vi "Weather Parse Test.vi"() -> ()   [LabVIEW 2020, in "CDM-Config.lvlib"] (continued)
\"2025-12-02T17:12:00-07:00\"\n                    }\n                ],\n                \"sent\": \"2025-12-03T02:08:00-07:00\",\n                \"effective\": \"2025-12-03T02:08:00-07:00\",\n                \"onset\": \"2025-12-03T02:08:00-07:00\",\n                \"expires\": \"2025-12-03T17:00:00-07:00\",\n                \"ends\": \"2025-12-04T02:00:00-07:00\",\n                \"status\": \"Actual\",\n                \"messageType\": \"Update\",\n                \"category\": \"Met\",\n                \"severity\": \"Moderate\",\n                \"certainty\": \"Likely\",\n                \"urgency\": \"Expected\",\n                \"event\": \"Winter Weather Advisory\",\n                \"sender\": \"w-nws.webmaster@noaa.gov\",\n                \"senderName\": \"NWS Grand Junction CO\",\n                \"headline\": \"Winter Weather Advisory issued December 3 at 2:08AM MST until December 4 at 2:00AM MST by NWS Grand Junction CO\",\n                \"description\": \"* WHAT...Snow. Total snow accumulations between 6 and 10 inches with\\nlocally higher amounts.\\n\\n* WHERE...Southwest San Juan Mountains.\\n\\n* WHEN...Until 2 AM MST Thursday.\\n\\n* IMPACTS...Travel could be very difficult. The hazardous conditions\\ncould impact the Wednesday morning and evening commutes.\",\n                \"instruction\": \"Slow down and use caution while traveling. The latest road\\nconditions for the state you are calling from can be obtained by\\ncalling 5 1 1.\",\n                \"response\": \"Execute\",\n                \"parameters\": {\n                    \"AWIPSidentifier\": [\n                        \"WSWGJT\"\n                    ],\n                    \"WMOidentifier\": [\n                        \"WWUS45 KGJT 030908\"\n                    ],\n                    \"NWSheadline\": [\n                        \"WINTER WEATHER ADVISORY REMAINS IN EFFECT UNTIL 2 AM MST THURSDAY\"\n                    ],\n                    \"BLOCKCHANNEL\": [\n                        \"EAS\",\n                        \"NWEM\",\n                        \"CMAS\"\n                    ],\n                    \"VTEC\": [\n                        \"/O.CON.KGJT.WW.Y.0026.000000T0000Z-251204T0900Z/\"\n                    ],\n                    \"eventEndingTime\": [\n                        \"2025-12-04T02:00:00-07:00\"\n                    ]\n                },\n                \"scope\": \"Public\",\n                \"code\": \"IPAWSv1.0\",\n                \"language\": \"en-US\",\n                \"web\": \"http://www.weather.gov\",\n                \"eventCode\": {\n                    \"SAME\": [\n                        \"NWS\"\n                    ],\n                    \"NationalWeatherService\": [\n                        \"WWY\"\n                    ]\n                }\n            }\n        },\n        {\n            \"id\": \"https://api.weather.gov/alerts/urn:oid:2.49.0.1.840.0.ecc18ad1715ddd59d073d3396e68cd94d8156f26.002.1\",\n            \"type\": \"Feature\",\n            \"geometry\": null,\n            \"properties\": {\n                \"@id\": \"https://api.weather.gov/alerts/urn:oid:2.49.0.1.840.0.ecc18ad1715ddd59d073d3396e68cd94d8156f26.002.1\",\n                \"@type\": \"wx:Alert\",\n                \"id\": \"urn:oid:2.49.0.1.840.0.ecc18ad1715ddd59d073d3396e68cd94d8156f26.002.1\",\n                \"areaDesc\": \"Elkhead and Park Mountains; Gore and Elk Mountains/Central Mountain Valleys\",\n                \"geocode\": {\n                    \"SAME\": [\n                        \"008081\",\n                        \"008107\",\n                        \"008037\",\n                        \"008045\",\n                        \"008097\"\n                    ],\n                    \"UGC\": [\n                        \"COZ004\",\n                        \"COZ010\"\n                    ]\n                },\n                \"affectedZones\": [\n                    \"https://api.weather.gov/zones/forecast/COZ004\",\n                    \"https://api.weather.gov/zones/forecast/COZ010\"\n                ],\n                \"references\": [\n                    {\n                        \"@id\": \"https://api.weather.gov/alerts/urn:oid:2.49.0.1.840.0.59f7bbb1b05f341c96e55d508e395b781ba80eb6.003.1\",\n                        \"identifier\": \"urn:oid:2.49.0.1.840.0.59f7bbb1b05f341c96e55d508e395b781ba80eb6.003.1\",\n                        \"sender\": \"w-nws.webmaster@noaa.gov\",\n                        \"sent\": \"2025-12-02T12:59:00-07:00\"\n                    },\n                    {\n                        \"@id\": \"https://api.weather.gov/alerts/urn:oid:2.49.0.1.840.0.1e2e3f318117076bbf552163bdfe24a72a2e2d99.002.1\",\n                        \"identifier\": \"urn:oid:2.49.0.1.840.0.1e2e3f318117076bbf552163bdfe24a72a2e2d99.002.1\",\n                        \"sender\": \"w-nws.webmaster@noaa.gov\",\n                        \"sent\": \"2025-12-02T17:12:00-07:00\"\n                    }\n                ],\n                \"sent\": \"2025-12-03T02:08:00-07:00\",\n                \"effective\": \"2025-12-03T02:08:00-07:00\",\n                \"onset\": \"2025-12-03T02:08:00-07:00\",\n                \"expires\": \"2025-12-03T17:00:00-07:00\",\n                \"ends\": \"2025-12-03T17:00:00-07:00\",\n                \"status\": \"Actual\",\n                \"messageType\": \"Update\",\n                \"category\": \"Met\",\n                \"severity\": \"Moderate\",\n                \"certainty\": \"Likely\",\n                \"urgency\": \"Expected\",\n                \"event\": \"Winter Weather Advisory\",\n                \"sender\": \"w-nws.webmaster@noaa.gov\",\n                \"senderName\": \"NWS Grand Junction CO\",\n                \"headline\": \"Winter Weather Advisory issued December 3 at 2:08AM MST until December 3 at 5:00PM MST by NWS Grand Junction CO\",\n                \"description\": \"* WHAT...Snow. Additional snow accumulations between 2 and 4 inches.\\n\\n* WHERE...Elkhead and Park Mountains, Northwest San Juan Mountains,\\nand Gore and Elk Mountains/Central Mountain Valleys.\\n\\n* WHEN...Until 5 PM MST this afternoon.\\n\\n* IMPACTS...Roads, and especially bridges and overpasses, will\\nlikely become slick and hazardous. Plan on slippery road\\nconditions. The hazardous conditions could impact the Wednesday\\nmorning and evening commutes.\",\n                \"instruction\": \"Slow down and use caution while traveling. The latest road\\nconditions for the state you are calling from can be obtained by\\ncalling 5 1 1.\",\n                \"response\": \"Execute\",\n                \"parameters\": {\n                    \"AWIPSidentifier\": [\n                        \"WSWGJT\"\n                    ],\n                    \"WMOidentifier\": [\n                        \"WWUS45 KGJT 030908\"\n                    ],\n                    \"NWSheadline\": [\n                        \"WINTER WEATHER ADVISORY REMAINS IN EFFECT UNTIL 5 PM MST THIS AFTERNOON\"\n                    ],\n                    \"BLOCKCHANNEL\": [\n                        \"EAS\",\n                        \"NWEM\",\n                        \"CMAS\"\n                    ],\n                    \"VTEC\": [\n                        \"/O.CON.KGJT.WW.Y.0026.000000T0000Z-251204T0000Z/\"\n                    ],\n                    \"eventEndingTime\": [\n                        \"2025-12-03T17:00:00-07:00\"\n                    ],\n                    \"expiredReferences\": [\n                        \"w-nws.webmaster@noaa.gov,urn:oid:2.49.0.1.840.0.679f6cdd98833ec879584b0a7abc7307ca2a58e6.001.1,2025-12-02T02:26:00-07:00\"\n                    ]\n                },\n                \"scope\": \"Public\",\n                \"code\": \"IPAWSv1.0\",\n                \"language\": \"en-US\",\n                \"web\": \"http://www.weather.gov\",\n                \"eventCode\": {\n                    \"SAME\": [\n                        \"NWS\"\n                    ],\n                    \"NationalWeatherService\": [\n                        \"WWY\"\n                    ]\n                }\n            }\n        },\n        {\n            \"id\": \"https://api.weather.gov/alerts/urn:oid:2.49.0.1.840.0.ecc18ad1715ddd59d073d3396e68cd94d8156f26.004.1\",\n            \"type\": \"Feature\",\n            \"geometry\": null,\n            \"properties\": {\n                \"@id\": \"https://api.weather.gov/alerts/urn:oid:2.49.0.1.840.0.ecc18ad1715ddd59d073d3396e68cd94d8156f26.004.1\",\n                \"@type\": \"wx:Alert\",\n                \"id\": \"urn:oid:2.49.0.1.840.0.ecc18ad1715ddd59d073d3396e68cd94d8156f26.004.1\",\n                \"areaDesc\": \"Northwestern San Juan Mountains\",\n                \"geocode\": {\n                    \"SAME\": [\n                        \"008051\",\n                        \"008053\",\n                        \"008085\",\n                        \"008091\",\n                        \"008113\"\n                    ],\n                    \"UGC\": [\n                        \"COZ018\"\n                    ]\n                },\n                \"affectedZones\": [\n                    \"https://api.weather.gov/zones/forecast/COZ018\"\n                ],\n                \"references\": [\n                    {\n                        \"@id\": \"https://api.weather.gov/alerts/urn:oid:2.49.0.1.840.0.59f7bbb1b05f341c96e55d508e395b781ba80eb6.002.1\",\n                        \"identifier\": \"urn:oid:2.49.0.1.840.0.59f7bbb1b05f341c96e55d508e395b781ba80eb6.002.1\",\n                        \"sender\": \"w-nws.webmaster@noaa.gov\",\n                        \"sent\": \"2025-12-02T12:59:00-07:00\"\n                    },\n                    {\n                        \"@id\": \"https://api.weather.gov/alerts/urn:oid:2.49.0.1.840.0.1e2e3f318117076bbf552163bdfe24a72a2e2d99.003.1\",\n                        \"identifier\": \"urn:oid:2.49.0.1.840.0.1e2e3f318117076bbf552163bdfe24a72a2e2d99.003.1\",\n                        \"sender\": \"w-nws.webmaster@noaa.gov\",\n                        \"sent\": \"2025-12-02T17:12:00-07:00\"\n                    }\n                ],\n                \"sent\": \"2025-12-03T02:08:00-07:00\",\n                \"effective\": \"2025-12-03T02:08:00-07:00\",\n                \"onset\": \"2025-12-03T02:08:00-07:00\",\n                \"expires\": \"2025-12-03T17:00:00-07:00\",\n                \"ends\": \"2025-12-04T02:00:00-07:00\",\n                \"status\": \"Actual\",\n                \"messageType\": \"Update\",\n                \"category\": \"Met\",\n                \"severity\": \"Moderate\",\n                \"certainty\": \"Likely\",\n                \"urgency\": \"Expected\",\n                \"event\": \"Winter Weather Advisory\",\n                \"sender\": \"w-nws.webmaster@noaa.gov\",\n                \"senderName\": \"NWS Grand Junction CO\",\n                \"headline\": \"Winter Weather Advisory issued December 3 at 2:08AM MST until December 4 at 2:00AM MST by NWS Grand Junction CO\",\n                \"description\": \"* WHAT...Snow. Total snow accumulations between 6 and 10 inches with\\nlocally higher amounts.\\n\\n* WHERE...Northwest San Juan Mountains.\\n\\n* WHEN...Until 2 AM MST Thursday.\\n\\n* IMPACTS...Travel could be very difficult. The hazardous conditions\\ncould impact the Wednesday morning and evening commutes.\",\n                \"instruction\": \"Slow down and use caution while traveling. The latest road\\nconditions for the state you are calling from can be obtained by\\ncalling 5 1 1.\",\n                \"response\": \"Execute\",\n                \"parameters\": {\n                    \"AWIPSidentifier\": [\n                        \"WSWGJT\"\n                    ],\n                    \"WMOidentifier\": [\n                        \"WWUS45 KGJT 030908\"\n                    ],\n                    \"NWSheadline\": [\n                        \"WINTER WEATHER ADVISORY REMAINS IN EFFECT UNTIL 2 AM MST THURSDAY\"\n                    ],\n                    \"BLOCKCHANNEL\": [\n                        \"EAS\",\n                        \"NWEM\",\n                        \"CMAS\"\n                    ],\n                    \"VTEC\": [\n                        \"/O.CON.KGJT.WW.Y.0026.000000T0000Z-251204T0900Z/\"\n                    ],\n                    \"eventEndingTime\": [\n                        \"2025-12-04T02:00:00-07:00\"\n                    ],\n                    \"expiredReferences\": [\n                        \"w-nws.webmaster@noaa.gov,urn:oid:2.49.0.1.840.0.679f6cdd98833ec879584b0a7abc7307ca2a58e6.001.1,2025-12-02T02:26:00-07:00\"\n                    ]\n                },\n                \"scope\": \"Public\",\n                \"code\": \"IPAWSv1.0\",\n                \"language\": \"en-US\",\n                \"web\": \"http://www.weather.gov\",\n                \"eventCode\": {\n                    \"SAME\": [\n                        \"NWS\"\n                    ],\n                    \"NationalWeatherService\": [\n                        \"WWY\"\n                    ]\n                }\n            }\n        },\n        {\n            \"id\": \"https://api.weather.gov/alerts/urn:oid:2.49.0.1.840.0.e71cf2b83fde77384319b715682951004f37611d.001.2\",\n            \"type\": \"Feature\",\n            \"geometry\": null,\n            \"properties\": {\n                \"@id\": \"https://api.weather.gov/alerts/urn:oid:2.49.0.1.840.0.e71cf2b83fde77384319b715682951004f37611d.001.2\",\n                \"@type\": \"wx:Alert\",\n                \"id\": \"urn:oid:2.49.0.1.840.0.e71cf2b83fde77384319b715682951004f37611d.001.2\",\n                \"areaDesc\": \"Rock Island Passage to Sturgeon Bay WI\",\n                \"geocode\": {\n                    \"SAME\": [\n                        \"092541\"\n                    ],\n                    \"UGC\": [\n                        \"LMZ541\"\n                    ]\n                },\n                \"affectedZones\": [\n                    \"https://api.weather.gov/zones/forecast/LMZ541\"\n                ],\n                \"references\": [],\n                \"sent\": \"2025-12-03T03:06:00-06:00\",\n                \"effective\": \"2025-12-03T03:06:00-06:00\",\n                \"onset\": \"2025-12-04T21:00:00-06:00\",\n                \"expires\": \"2025-12-03T11:15:00-06:00\",\n                \"ends\": \"2025-12-05T06:00:00-06:00\",\n                \"status\": \"Actual\",\n                \"messageType\": \"Alert\",\n                \"category\": \"Met\",\n                \"severity\": \"Moderate\",\n                \"certainty\": \"Possible\",\n                \"urgency\": \"Future\",\n                \"event\": \"Gale Watch\",\n                \"sender\": \"w-nws.webmaster@noaa.gov\",\n                \"senderName\": \"NWS Green Bay WI\",\n                \"headline\": \"Gale Watch issued December 3 at 3:06AM CST until December 5 at 6:00AM CST by NWS Green Bay WI\",\n                \"description\": \"* WHAT...For the Small Craft Advisory, northwest winds 15 to 20\\nkt with gusts up to 25 kt and waves 2 to 5 ft. For the Gale\\nWatch, southwest winds 20 to 25 kt with gusts up to 35 kt and\\nwaves 4 to 7 ft possible.\\n\\n* WHERE...Lake Michigan nearshore waters from Washington Island\\nto Sturgeon Bay.\\n\\n* WHEN...For the Small Craft Advisory, until 3 AM CST Thursday.\\nFor the Gale Watch, from Thursday evening through late\\nThursday night.\\n\\n* IMPACTS...Strong winds can cause hazardous waves which could\\ncapsize or damage vessels and reduce visibility.\",\n                \"instruction\": \"Mariners should consider altering plans to avoid possible\\nhazardous conditions.  Remain in port, seek safe harbor, alter\\ncourse, and/or secure the vessel for severe wind and waves.\",\n                \"response\": \"Prepare\",\n                \"parameters\": {\n                    \"AWIPSidentifier\": [\n                        \"MWWGRB\"\n                    ],\n                    \"WMOidentifier\": [\n                        \"WHUS73 KGRB 030906\"\n                    ],\n                    \"NWSheadline\": [\n                        \"SMALL CRAFT ADVISORY REMAINS IN EFFECT UNTIL 3 AM CST THURSDAY... ...GALE WATCH IN EFFECT FROM THURSDAY EVENING THROUGH LATE THURSDAY NIGHT\"\n                    ],\n                    \"BLOCKCHANNEL\": [\n                        \"EAS\",\n                        \"NWEM\",\n                        \"CMAS\"\n                    ],\n                    \"VTEC\": [\n                        \"/O.NEW.KGRB.GL.A.0006.251205T0300Z-251205T1200Z/\"\n                    ],\n                    \"eventEndingTime\": [\n                        \"2025-12-05T06:00:00-06:00\"\n                    ]\n                },\n                \"scope\": \"Public\",\n                \"code\": \"IPAWSv1.0\",\n                \"language\": \"en-US\",\n                \"web\": \"http://www.weather.gov\",\n                \"eventCode\": {\n                    \"SAME\": [\n                        \"NWS\"\n                    ],\n                    \"NationalWeatherService\": [\n                        \"GLA\"\n                    ]\n                }\n            }\n        },\n        {\n            \"id\": \"https://api.weather.gov/alerts/urn:oid:2.49.0.1.840.0.e71cf2b83fde77384319b715682951004f37611d.002.2\",\n            \"type\": \"Feature\",\n            \"geometry\": null,\n            \"properties\": {\n                \"@id\": \"https://api.weather.gov/alerts/urn:oid:2.49.0.1.840.0.e71cf2b83fde77384319b715682951004f37611d.002.2\",\n                \"@type\": \"wx:Alert\",\n                \"id\": \"urn:oid:2.49.0.1.840.0.e71cf2b83fde77384319b715682951004f37611d.002.2\",\n                \"areaDesc\": \"Green Bay south of line from  Cedar River to Rock Island Passage and north of a line from Oconto WI to Little Sturgeon Bay WI\",\n                \"geocode\": {\n                    \"SAME\": [\n                        \"092521\"\n                    ],\n                    \"UGC\": [\n                        \"LMZ521\"\n                    ]\n                },\n                \"affectedZones\": [\n                    \"https://api.weather.gov/zones/forecast/LMZ521\"\n                ],\n                \"references\": [],\n                \"sent\": \"2025-12-03T03:06:00-06:00\",\n                \"effective\": \"2025-12-03T03:06:00-06:00\",\n                \"onset\": \"2025-12-04T21:00:00-06:00\",\n                \"expires\": \"2025-12-03T11:15:00-06:00\",\n                \"ends\": \"2025-12-05T06:00:00-06:00\",\n                \"status\": \"Actual\",\n                \"messageType\": \"Alert\",\n                \"category\": \"Met\",\n                \"severity\": \"Moderate\",\n                \"certainty\": \"Possible\",\n                \"urgency\": \"Future\",\n                \"event\": \"Gale Watch\",\n                \"sender\": \"w-nws.webmaster@noaa.gov\",\n                \"senderName\": \"NWS Green Bay WI\",\n                \"headline\": \"Gale Watch issued December 3 at 3:06AM CST until December 5 at 6:00AM CST by NWS Green Bay WI\",\n                \"description\": \"* WHAT...For the Small Craft Advisory, northwest winds 15 to 25\\nkt and waves 1 to 4 ft. For the Gale Watch, southwest winds 20\\nto 25 kt with gusts up to 35 kt and waves 5 to 8 ft possible.\\n\\n* WHERE...Central Bay of Green Bay.\\n\\n* WHEN...For the Small Craft Advisory, until 3 AM CST Thursday.\\nFor the Gale Watch, from Thursday evening through late\\nThursday night.\\n\\n* IMPACTS...Strong winds can cause hazardous waves which could\\ncapsize or damage vessels and reduce visibility.\",\n                \"instruction\": \"Mariners should consider altering plans to avoid possible\\nhazardous conditions.  Remain in port, seek safe harbor, alter\\ncourse, and/or secure the vessel for severe wind and waves.\",\n                \"response\": \"Prepare\",\n                \"parameters\": {\n                    \"AWIPSidentifier\": [\n                        \"MWWGRB\"\n                    ],\n                    \"WMOidentifier\": [\n                        \"WHUS73 KGRB 030906\"\n                    ],\n                    \"NWSheadline\": [\n                        \"SMALL CRAFT ADVISORY REMAINS IN EFFECT UNTIL 3 AM CST THURSDAY... ...GALE WATCH IN EFFECT FROM THURSDAY EVENING THROUGH LATE THURSDAY NIGHT\"\n                    ],\n                    \"BLOCKCHANNEL\": [\n                        \"EAS\",\n                        \"NWEM\",\n                        \"CMAS\"\n                    ],\n                    \"VTEC\": [\n                        \"/O.NEW.KGRB.GL.A.0006.251205T0300Z-251205T1200Z/\"\n                    ],\n                    \"eventEndingTime\": [\n                        \"2025-12-05T06:00:00-06:00\"\n                    ]\n                },\n                \"scope\": \"Public\",\n                \"code\": \"IPAWSv1.0\",\n                \"language\": \"en-US\",\n                \"web\": \"http://www.weather.gov\",\n                \"eventCode\": {\n                    \"SAME\": [\n                        \"NWS\"\n                    ],\n                    \"NationalWeatherService\": [\n                        \"GLA\"\n                    ]\n                }\n            }\n        },\n        {\n            \"id\": \"https://api.weather.gov/alerts/urn:oid:2.49.0.1.840.0.e71cf2b83fde77384319b715682951004f37611d.002.1\",\n            \"type\": \"Feature\",\n            \"geometry\": null,\n            \"properties\": {\n                \"@id\": \"https://api.weather.gov/alerts/urn:oid:2.49.0.1.840.0.e71cf2b83fde77384319b715682951004f37611d.002.1\",\n                \"@type\": \"wx:Alert\",\n                \"id\": \"urn:oid:2.49.0.1.840.0.e71cf2b83fde77384319b715682951004f37611d.002.1\",\n                \"areaDesc\": \"Green Bay south of line from  Cedar River to Rock Island Passage and north of a line from Oconto WI to Little Sturgeon Bay WI\",\n                \"geocode\": {\n                    \"SAME\": [\n                        \"092521\"\n                    ],\n                    \"UGC\": [\n                        \"LMZ521\"\n                    ]\n                },\n                \"affectedZones\": [\n                    \"https://api.weather.gov/zones/forecast/LMZ521\"\n                ],\n                \"references\": [\n                    {\n                        \"@id\": \"https://api.weather.gov/alerts/urn:oid:2.49.0.1.840.0.769b5a057bb88d56f701a5e0b04efae8c3b52336.002.1\",\n                        \"identifier\": \"urn:oid:2.49.0.1.840.0.769b5a057bb88d56f701a5e0b04efae8c3b52336.002.1\",\n                        \"sender\": \"w-nws.webmaster@noaa.gov\",\n                        \"sent\": \"2025-12-02T21:04:00-06:00\"\n                    }\n                ],\n                \"sent\": \"2025-12-03T03:06:00-06:00\",\n                \"effective\": \"2025-12-03T03:06:00-06:00\",\n                \"onset\": \"2025-12-03T03:06:00-06:00\",\n                \"expires\": \"2025-12-03T11:15:00-06:00\",\n                \"ends\": \"2025-12-04T03:00:00-06:00\",\n                \"status\": \"Actual\",\n                \"messageType\": \"Update\",\n                \"category\": \"Met\",\n                \"severity\": \"Minor\",\n                \"certainty\": \"Likely\",\n                \"urgency\": \"Expected\",\n                \"event\": \"Small Craft Advisory\",\n                \"sender\": \"w-nws.webmaster@noaa.gov\",\n                \"senderName\": \"NWS Green Bay WI\",\n                \"headline\": \"Small Craft Advisory issued December 3 at 3:06AM CST until December 4 at 3:00AM CST by NWS Green Bay WI\",\n                \"description\": \"* WHAT...For the Small Craft Advisory, northwest winds 15 to 25\\nkt and waves 1 to 4 ft. For the Gale Watch, southwest winds 20\\nto 25 kt with gusts up to 35 kt and waves 5 to 8 ft possible.\\n\\n* WHERE...Central Bay of Green Bay.\\n\\n* WHEN...For the Small Craft Advisory, until 3 AM CST Thursday.\\nFor the Gale Watch, from Thursday evening through late\\nThursday night.\\n\\n* IMPACTS...Strong winds can cause hazardous waves which could\\ncapsize or damage vessels and reduce visibility.\",\n                \"instruction\": \"Mariners should consider altering plans to avoid possible\\nhazardous conditions.  Remain in port, seek safe harbor, alter\\ncourse, and/or secure the vessel for severe wind and waves.\",\n                \"response\": \"Avoid\",\n                \"parameters\": {\n                    \"AWIPSidentifier\": [\n                        \"MWWGRB\"\n                    ],\n                    \"WMOidentifier\": [\n                        \"WHUS73 KGRB 030906\"\n                    ],\n                    \"NWSheadline\": [\n                        \"SMALL CRAFT ADVISORY REMAINS IN EFFECT UNTIL 3 AM CST THURSDAY... ...GALE WATCH IN EFFECT FROM THURSDAY EVENING THROUGH LATE THURSDAY NIGHT\"\n                    ],\n                    \"BLOCKCHANNEL\": [\n                        \"EAS\",\n                        \"NWEM\",\n                        \"CMAS\"\n                    ],\n                    \"VTEC\": [\n                        \"/O.CON.KGRB.SC.Y.0092.000000T0000Z-251204T0900Z/\"\n                    ],\n                    \"eventEndingTime\": [\n                        \"2025-12-04T03:00:00-06:00\"\n                    ],\n                    \"expiredReferences\": [\n                        \"w-nws.webmaster@noaa.gov,urn:oid:2.49.0.1.840.0.4daec37cfaba31be0f4161c4db8c289fd8fca270.002.1,2025-12-02T16:20:00-06:00 w-nws.webmaster@noaa.gov,urn:oid:2.49.0.1.840.0.22088d8fd19601efe26ef283f0aea20a6c82bd22.002.1,2025-12-02T10:40:00-06:00 w-nws.webmaster@noaa.gov,urn:oid:2.49.0.1.840.0.4d26ff1add25a90f0bbaf88a1a22cd2917cf1fd9.002.1,2025-12-02T03:00:00-06:00\"\n                    ]\n                },\n                \"scope\": \"Public\",\n                \"code\": \"IPAWSv1.0\",\n                \"language\": \"en-US\",\n                \"web\": \"http://www.weather.gov\",\n                \"eventCode\": {\n                    \"SAME\": [\n                        \"NWS\"\n                    ],\n                    \"NationalWeatherService\": [\n                        \"SCY\"\n                    ]\n                }\n            }\n        },\n        {\n            \"id\": \"https://api.weather.gov/alerts/urn:oid:2.49.0.1.840.0.e71cf2b83fde77384319b715682951004f37611d.004.1\",\n            \"type\": \"Feature\",\n            \"geometry\": null,\n            \"properties\": {\n                \"@id\": \"https://api.weather.gov/alerts/urn:oid:2.49.0.1.840.0.e71cf2b83fde77384319b715682951004f37611d.004.1\",\n                \"@type\": \"wx:Alert\",\n                \"id\": \"urn:oid:2.49.0.1.840.0.e71cf2b83fde77384319b715682951004f37611d.004.1\",\n                \"areaDesc\": \"Green Bay south of line from  Oconto WI to Little Sturgeon Bay WI\",\n                \"geocode\": {\n                    \"SAME\": [\n                        \"092522\"\n                    ],\n                    \"UGC\": [\n                        \"LMZ522\"\n                    ]\n                },\n                \"affectedZones\": [\n                    \"https://api.weather.gov/zones/forecast/LMZ522\"\n                ],\n                \"references\": [\n                    {\n                        \"@id\": \"https://api.weather.gov/alerts/urn:oid:2.49.0.1.840.0.769b5a057bb88d56f701a5e0b04efae8c3b52336.002.1\",\n                        \"identifier\": \"urn:oid:2.49.0.1.840.0.769b5a057bb88d56f701a5e0b04efae8c3b52336.002.1\",\n                        \"sender\": \"w-nws.webmaster@noaa.gov\",\n                        \"sent\": \"2025-12-02T21:04:00-06:00\"\n                    }\n                ],\n                \"sent\": \"2025-12-03T03:06:00-06:00\",\n                \"effective\": \"2025-12-03T03:06:00-06:00\",\n                \"onset\": \"2025-12-03T03:06:00-06:00\",\n                \"expires\": \"2025-12-03T11:15:00-06:00\",\n                \"ends\": \"2025-12-04T03:00:00-06:00\",\n                \"status\": \"Actual\",\n                \"messageType\": \"Update\",\n                \"category\": \"Met\",\n                \"severity\": \"Minor\",\n                \"certainty\": \"Likely\",\n                \"urgency\": \"Expected\",\n                \"event\": \"Small Craft Advisory\",\n                \"sender\": \"w-nws.webmaster@noaa.gov\",\n                \"senderName\": \"NWS Green Bay WI\",\n                \"headline\": \"Small Craft Advisory issued December 3 at 3:06AM CST until December 4 at 3:00AM CST by NWS Green Bay WI\",\n                \"description\": \"* WHAT...Northwest winds 15 to 25 kt and waves 1 to 3 ft.\\n\\n* WHERE...Southern Bay of Green Bay.\\n\\n* WHEN...Until 3 AM CST Thursday.\\n\\n* IMPACTS...Conditions will be hazardous to small craft.\",\n                \"instruction\": \"Inexperienced mariners, especially those operating smaller\\nvessels, should avoid navigating in hazardous conditions.\",\n                \"response\": \"Avoid\",\n                \"parameters\": {\n                    \"AWIPSidentifier\": [\n                        \"MWWGRB\"\n                    ],\n                    \"WMOidentifier\": [\n                        \"WHUS73 KGRB 030906\"\n                    ],\n                    \"NWSheadline\": [\n                        \"SMALL CRAFT ADVISORY REMAINS IN EFFECT UNTIL 3 AM CST THURSDAY\"\n                    ],\n                    \"BLOCKCHANNEL\": [\n                        \"EAS\",\n                        \"NWEM\",\n                        \"CMAS\"\n                    ],\n                    \"VTEC\": [\n                        \"/O.CON.KGRB.SC.Y.0092.000000T0000Z-251204T0900Z/\"\n                    ],\n                    \"eventEndingTime\": [\n                        \"2025-12-04T03:00:00-06:00\"\n                    ],\n                    \"expiredReferences\": [\n                        \"w-nws.webmaster@noaa.gov,urn:oid:2.49.0.1.840.0.4daec37cfaba31be0f4161c4db8c289fd8fca270.002.1,2025-12-02T16:20:00-06:00 w-nws.webmaster@noaa.gov,urn:oid:2.49.0.1.840.0.22088d8fd19601efe26ef283f0aea20a6c82bd22.002.1,2025-12-02T10:40:00-06:00 w-nws.webmaster@noaa.gov,urn:oid:2.49.0.1.840.0.4d26ff1add25a90f0bbaf88a1a22cd2917cf1fd9.002.1,2025-12-02T03:00:00-06:00\"\n                    ]\n                },\n                \"scope\": \"Public\",\n                \"code\": \"IPAWSv1.0\",\n                \"language\": \"en-US\",\n                \"web\": \"http://www.weather.gov\",\n                \"eventCode\": {\n                    \"SAME\": [\n                        \"NWS\"\n                    ],\n                    \"NationalWeatherService\": [\n                        \"SCY\"\n                    ]\n                }\n            }\n        },\n        {\n            \"id\": \"https://api.weather.gov/alerts/urn:oid:2.49.0.1.840.0.e71cf2b83fde77384319b715682951004f37611d.001.1\",\n            \"type\": \"Feature\",\n            \"geometry\": null,\n            \"properties\": {\n                \"@id\": \"https://api.weather.gov/alerts/urn:oid:2.49.0.1.840.0.e71cf2b83fde77384319b715682951004f37611d.001.1\",\n                \"@type\": \"wx:Alert\",\n                \"id\": \"urn:oid:2.49.0.1.840.0.e71cf2b83fde77384319b715682951004f37611d.001.1\",\n                \"areaDesc\": \"Rock Island Passage to Sturgeon Bay WI\",\n                \"geocode\": {\n                    \"SAME\": [\n                        \"092541\"\n                    ],\n                    \"UGC\": [\n                        \"LMZ541\"\n                    ]\n                },\n                \"affectedZones\": [\n                    \"https://api.weather.gov/zones/forecast/LMZ541\"\n                ],\n                \"references\": [\n                    {\n                        \"@id\": \"https://api.weather.gov/alerts/urn:oid:2.49.0.1.840.0.769b5a057bb88d56f701a5e0b04efae8c3b52336.001.1\",\n                        \"identifier\": \"urn:oid:2.49.0.1.840.0.769b5a057bb88d56f701a5e0b04efae8c3b52336.001.1\",\n                        \"sender\": \"w-nws.webmaster@noaa.gov\",\n                        \"sent\": \"2025-12-02T21:04:00-06:00\"\n                    }\n                ],\n                \"sent\": \"2025-12-03T03:06:00-06:00\",\n                \"effective\": \"2025-12-03T03:06:00-06:00\",\n                \"onset\": \"2025-12-03T03:06:00-06:00\",\n                \"expires\": \"2025-12-03T11:15:00-06:00\",\n                \"ends\": \"2025-12-04T03:00:00-06:00\",\n                \"status\": \"Actual\",\n                \"messageType\": \"Update\",\n                \"category\": \"Met\",\n                \"severity\": \"Minor\",\n                \"certainty\": \"Likely\",\n                \"urgency\": \"Expected\",\n                \"event\": \"Small Craft Advisory\",\n                \"sender\": \"w-nws.webmaster@noaa.gov\",\n                \"senderName\": \"NWS Green Bay WI\",\n                \"headline\": \"Small Craft Advisory issued December 3 at 3:06AM CST until December 4 at 3:00AM CST by NWS Green Bay WI\",\n                \"description\": \"* WHAT...For the Small Craft Advisory, northwest winds 15 to 20\\nkt with gusts up to 25 kt and waves 2 to 5 ft. For the Gale\\nWatch, southwest winds 20 to 25 kt with gusts up to 35 kt and\\nwaves 4 to 7 ft possible.\\n\\n* WHERE...Lake Michigan nearshore waters from Washington Island\\nto Sturgeon Bay.\\n\\n* WHEN...For the Small Craft Advisory, until 3 AM CST Thursday.\\nFor the Gale Watch, from Thursday evening through late\\nThursday night.\\n\\n* IMPACTS...Strong winds can cause hazardous waves which could\\ncapsize or damage vessels and reduce visibility.\",\n                \"instruction\": \"Mariners should consider altering plans to avoid possible\\nhazardous conditions.  Remain in port, seek safe harbor, alter\\ncourse, and/or secure the vessel for severe wind and waves.\",\n                \"response\": \"Avoid\",\n                \"parameters\": {\n                    \"AWIPSidentifier\": [\n                        \"MWWGRB\"\n                    ],\n                    \"WMOidentifier\": [\n                        \"WHUS73 KGRB 030906\"\n                    ],\n                    \"NWSheadline\": [\n                        \"SMALL CRAFT ADVISORY REMAINS IN EFFECT UNTIL 3 AM CST THURSDAY... ...GALE WATCH IN EFFECT FROM THURSDAY EVENING THROUGH LATE THURSDAY NIGHT\"\n                    ],\n                    \"BLOCKCHANNEL\": [\n                        \"EAS\",\n                        \"NWEM\",\n                        \"CMAS\"\n                    ],\n                    \"VTEC\": [\n                        \"/O.CON.KGRB.SC.Y.0092.000000T0000Z-251204T0900Z/\"\n                    ],\n                    \"eventEndingTime\": [\n                        \"2025-12-04T03:00:00-06:00\"\n                    ],\n                    \"expiredReferences\": [\n                        \"w-nws.webmaster@noaa.gov,urn:oid:2.49.0.1.840.0.4daec37cfaba31be0f4161c4db8c289fd8fca270.001.1,2025-12-02T16:20:00-06:00 w-nws.webmaster@noaa.gov,urn:oid:2.49.0.1.840.0.22088d8fd19601efe26ef283f0aea20a6c82bd22.001.1,2025-12-02T10:40:00-06:00 w-nws.webmaster@noaa.gov,urn:oid:2.49.0.1.840.0.4d26ff1add25a90f0bbaf88a1a22cd2917cf1fd9.001.1,2025-12-02T03:00:00-06:00\"\n                    ]\n                },\n                \"scope\": \"Public\",\n                \"code\": \"IPAWSv1.0\",\n                \"language\": \"en-US\",\n                \"web\": \"http://www.weather.gov\",\n                \"eventCode\": {\n                    \"SAME\": [\n                        \"NWS\"\n                    ],\n                    \"NationalWeatherService\": [\n                        \"SCY\"\n                    ]\n                }\n            }\n        },\n        {\n            \"id\": \"https://api.weather.gov/alerts/urn:oid:2.49.0.1.840.0.e71cf2b83fde77384319b715682951004f37611d.003.1\",\n            \"type\": \"Feature\",\n            \"geometry\": null,\n            \"properties\": {\n                \"@id\": \"https://api.weather.gov/alerts/urn:oid:2.49.0.1.840.0.e71cf2b83fde77384319b715682951004f37611d.003.1\",\n                \"@type\": \"wx:Alert\",\n                \"id\": \"urn:oid:2.49.0.1.840.0.e71cf2b83fde77384319b715682951004f37611d.003.1\",\n                \"areaDesc\": \"Sturgeon Bay to Two Rivers WI; Two Rivers to Sheboygan WI\",\n                \"geocode\": {\n                    \"SAME\": [\n                        \"092542\",\n                        \"092543\"\n                    ],\n                    \"UGC\": [\n                        \"LMZ542\",\n                        \"LMZ543\"\n                    ]\n                },\n                \"affectedZones\": [\n                    \"https://api.weather.gov/zones/forecast/LMZ542\",\n                    \"https://api.weather.gov/zones/forecast/LMZ543\"\n                ],\n                \"references\": [\n                    {\n                        \"@id\": \"https://api.weather.gov/alerts/urn:oid:2.49.0.1.840.0.769b5a057bb88d56f701a5e0b04efae8c3b52336.001.1\",\n                        \"identifier\": \"urn:oid:2.49.0.1.840.0.769b5a057bb88d56f701a5e0b04efae8c3b52336.001.1\",\n                        \"sender\": \"w-nws.webmaster@noaa.gov\",\n                        \"sent\": \"2025-12-02T21:04:00-06:00\"\n                    }\n                ],\n                \"sent\": \"2025-12-03T03:06:00-06:00\",\n                \"effective\": \"2025-12-03T03:06:00-06:00\",\n                \"onset\": \"2025-12-03T03:06:00-06:00\",\n                \"expires\": \"2025-12-03T11:15:00-06:00\",\n                \"ends\": \"2025-12-04T03:00:00-06:00\",\n                \"status\": \"Actual\",\n                \"messageType\": \"Update\",\n                \"category\": \"Met\",\n                \"severity\": \"Minor\",\n                \"certainty\": \"Likely\",\n                \"urgency\": \"Expected\",\n                \"event\": \"Small Craft Advisory\",\n                \"sender\": \"w-nws.webmaster@noaa.gov\",\n                \"senderName\": \"NWS Green Bay WI\",\n                \"headline\": \"Small Craft Advisory issued December 3 at 3:06AM CST until December 4 at 3:00AM CST by NWS Green Bay WI\",\n                \"description\": \"* WHAT...Northwest winds 15 to 20 kt with gusts up to 25 kt and\\nwaves 1 to 4 ft.\\n\\n* WHERE...Lake Michigan nearshore waters from Sturgeon Bay to\\nSheboygan.\\n\\n* WHEN...Until 3 AM CST Thursday.\\n\\n* IMPACTS...Conditions will be hazardous to small craft.\",\n                \"instruction\": \"Inexperienced mariners, especially those operating smaller\\nvessels, should avoid navigating in hazardous conditions.\",\n                \"response\": \"Avoid\",\n                \"parameters\": {\n                    \"AWIPSidentifier\": [\n                        \"MWWGRB\"\n                    ],\n                    \"WMOidentifier\": [\n                        \"WHUS73 KGRB 030906\"\n                    ],\n                    \"NWSheadline\": [\n                        \"SMALL CRAFT ADVISORY REMAINS IN EFFECT UNTIL 3 AM CST THURSDAY\"\n                    ],\n                    \"BLOCKCHANNEL\": [\n                        \"EAS\",\n                        \"NWEM\",\n                        \"CMAS\"\n                    ],\n                    \"VTEC\": [\n                        \"/O.CON.KGRB.SC.Y.0092.000000T0000Z-251204T0900Z/\"\n                    ],\n                    \"eventEndingTime\": [\n                        \"2025-12-04T03:00:00-06:00\"\n                    ],\n                    \"expiredReferences\": [\n                        \"w-nws.webmaster@noaa.gov,urn:oid:2.49.0.1.840.0.4daec37cfaba31be0f4161c4db8c289fd8fca270.001.1,2025-12-02T16:20:00-06:00 w-nws.webmaster@noaa.gov,urn:oid:2.49.0.1.840.0.22088d8fd19601efe26ef283f0aea20a6c82bd22.001.1,2025-12-02T10:40:00-06:00 w-nws.webmaster@noaa.gov,urn:oid:2.49.0.1.840.0.4d26ff1add25a90f0bbaf88a1a22cd2917cf1fd9.001.1,2025-12-02T03:00:00-06:00\"\n                    ]\n                },\n                \"scope\": \"Public\",\n                \"code\": \"IPAWSv1.0\",\n                \"language\": \"en-US\",\n                \"web\": \"http://www.weather.gov\",\n                \"eventCode\": {\n                    \"SAME\": [\n                        \"NWS\"\n                    ],\n                    \"NationalWeatherService\": [\n                        \"SCY\"\n                    ]\n                }\n            }\n        },\n        {\n            \"id\": \"https://api.weather.gov/alerts/urn:oid:2.49.0.1.840.0.32bbc1f07df14da85325353d729851465268ec74.002.1\",\n            \"type\": \"Feature\",\n            \"geometry\": null,\n            \"properties\": {\n                \"@id\": \"https://api.weather.gov/alerts/urn:oid:2.49.0.1.840.0.32bbc1f07df14da85325353d729851465268ec74.002.1\",\n                \"@type\": \"wx:Alert\",\n                \"id\": \"urn:oid:2.49.0.1.840.0.32bbc1f07df14da85325353d729851465268ec74.002.1\",\n                \"areaDesc\": \"Gary to Burns Harbor IN; Burns Harbor to Michigan City IN\",\n                \"geocode\": {\n                    \"SAME\": [\n                        \"092744\",\n                        \"092745\"\n                    ],\n                    \"UGC\": [\n                        \"LMZ744\",\n                        \"LMZ745\"\n                    ]\n                },\n                \"affectedZones\": [\n                    \"https://api.weather.gov/zones/forecast/LMZ744\",\n                    \"https://api.weather.gov/zones/forecast/LMZ745\"\n                ],\n                \"references\": [\n                    {\n                        \"@id\": \"https://api.weather.gov/alerts/urn:oid:2.49.0.1.840.0.0ae299528d7f4708a81affaa12e1a385ffcf6cb0.002.1\",\n                        \"identifier\": \"urn:oid:2.49.0.1.840.0.0ae299528d7f4708a81affaa12e1a385ffcf6cb0.002.1\",\n                        \"sender\": \"w-nws.webmaster@noaa.gov\",\n                        \"sent\": \"2025-12-02T21:56:00-06:00\"\n                    }\n                ],\n                \"sent\": \"2025-12-03T03:01:00-06:00\",\n                \"effective\": \"2025-12-03T03:01:00-06:00\",\n                \"onset\": \"2025-12-03T03:01:00-06:00\",\n                \"expires\": \"2025-12-03T11:15:00-06:00\",\n                \"ends\": \"2025-12-04T15:00:00-06:00\",\n                \"status\": \"Actual\",\n                \"messageType\": \"Update\",\n                \"category\": \"Met\",\n                \"severity\": \"Minor\",\n                \"certainty\": \"Likely\",\n                \"urgency\": \"Expected\",\n                \"event\": \"Small Craft Advisory\",\n                \"sender\": \"w-nws.webmaster@noaa.gov\",\n                \"senderName\": \"NWS Chicago IL\",\n                \"headline\": \"Small Craft Advisory issued December 3 at 3:01AM CST until December 4 at 3:00PM CST by NWS Chicago IL\",\n                \"description\": \"* WHAT...Southwest winds to 25 kt becoming northwest late this\\nafternoon. Significant waves to 9 ft occasionally to 12 ft.\\n\\n* WHERE...Gary to Michigan City IN.\\n\\n* WHEN...Until 3 PM CST Thursday.\\n\\n* IMPACTS...Conditions will be hazardous to small craft.\",\n                \"instruction\": \"Inexperienced mariners, especially those operating smaller\\nvessels, should avoid navigating in hazardous conditions.\",\n                \"response\": \"Avoid\",\n                \"parameters\": {\n                    \"AWIPSidentifier\": [\n                        \"MWWLOT\"\n                    ],\n                    \"WMOidentifier\": [\n                        \"WHUS73 KLOT 030901\"\n                    ],\n                    \"NWSheadline\": [\n                        \"SMALL CRAFT ADVISORY REMAINS IN EFFECT UNTIL 3 PM CST THURSDAY\"\n                    ],\n                    \"BLOCKCHANNEL\": [\n                        \"EAS\",\n                        \"NWEM\",\n                        \"CMAS\"\n                    ],\n                    \"VTEC\": [\n                        \"/O.CON.KLOT.SC.Y.0106.000000T0000Z-251204T2100Z/\"\n                    ],\n                    \"eventEndingTime\": [\n                        \"2025-12-04T15:00:00-06:00\"\n                    ],\n                    \"expiredReferences\": [\n                        \"w-nws.webmaster@noaa.gov,urn:oid:2.49.0.1.840.0.648f1635c62c08083c73378729536c6fc4072c7f.002.1,2025-12-02T15:03:00-06:00 w-nws.webmaster@noaa.gov,urn:oid:2.49.0.1.840.0.043c5ed733c295f69bb99c09650f0bff5bb0419a.002.1,2025-12-02T09:55:00-06:00 w-nws.webmaster@noaa.gov,urn:oid:2.49.0.1.840.0.d92e98cd2c5e6e07b963c8e6571b50d21b5478ee.002.1,2025-12-02T03:25:00-06:00\"\n                    ]\n                },\n                \"scope\": \"Public\",\n                \"code\": \"IPAWSv1.0\",\n                \"language\": \"en-US\",\n                \"web\": \"http://www.weather.gov\",\n                \"eventCode\": {\n                    \"SAME\": [\n                        \"NWS\"\n                    ],\n                    \"NationalWeatherService\": [\n                        \"SCY\"\n                    ]\n                }\n            }\n        },\n        {\n            \"id\": \"https://api.weather.gov/alerts/urn:oid:2.49.0.1.840.0.32bbc1f07df14da85325353d729851465268ec74.001.2\",\n            \"type\": \"Feature\",\n            \"geometry\": null,\n            \"properties\": {\n                \"@id\": \"https://api.weather.gov/alerts/urn:oid:2.49.0.1.840.0.32bbc1f07df14da85325353d729851465268ec74.001.2\",\n                \"@type\": \"wx:Alert\",\n                \"id\": \"urn:oid:2.49.0.1.840.0.32bbc1f07df14da85325353d729851465268ec74.001.2\",\n                \"areaDesc\": \"Winthrop Harbor to Wilmette Harbor IL; Wilmette Harbor to Northerly Island IL; Northerly Island to Calumet Harbor IL; Calumet Harbor IL to Gary IN\",\n                \"geocode\": {\n                    \"SAME\": [\n                        \"092740\",\n                        \"092741\",\n                        \"092742\",\n                        \"092743\"\n                    ],\n                    \"UGC\": [\n                        \"LMZ740\",\n                        \"LMZ741\",\n                        \"LMZ742\",\n                        \"LMZ743\"\n                    ]\n                },\n                \"affectedZones\": [\n                    \"https://api.weather.gov/zones/forecast/LMZ740\",\n                    \"https://api.weather.gov/zones/forecast/LMZ741\",\n                    \"https://api.weather.gov/zones/forecast/LMZ742\",\n                    \"https://api.weather.gov/zones/forecast/LMZ743\"\n                ],\n                \"references\": [\n                    {\n                        \"@id\": \"https://api.weather.gov/alerts/urn:oid:2.49.0.1.840.0.0ae299528d7f4708a81affaa12e1a385ffcf6cb0.001.2\",\n                        \"identifier\": \"urn:oid:2.49.0.1.840.0.0ae299528d7f4708a81affaa12e1a385ffcf6cb0.001.2\",\n                        \"sender\": \"w-nws.webmaster@noaa.gov\",\n                        \"sent\": \"2025-12-02T21:56:00-06:00\"\n                    }\n                ],\n                \"sent\": \"2025-12-03T03:01:00-06:00\",\n                \"effective\": \"2025-12-03T03:01:00-06:00\",\n                \"onset\": \"2025-12-03T21:00:00-06:00\",\n                \"expires\": \"2025-12-03T11:15:00-06:00\",\n                \"ends\": \"2025-12-04T09:00:00-06:00\",\n                \"status\": \"Actual\",\n                \"messageType\": \"Update\",\n                \"category\": \"Met\",\n                \"severity\": \"Minor\",\n                \"certainty\": \"Likely\",\n                \"urgency\": \"Expected\",\n                \"event\": \"Small Craft Advisory\",\n                \"sender\": \"w-nws.webmaster@noaa.gov\",\n                \"senderName\": \"NWS Chicago IL\",\n                \"headline\": \"Small Craft Advisory issued December 3 at 3:01AM CST until December 4 at 9:00AM CST by NWS Chicago IL\",\n                \"description\": \"* WHAT...For the first Small Craft Advisory, southwest winds to\\n25 kt and significant waves to 4 ft. For the second Small\\nCraft Advisory, northwest winds to 25 kt and significant waves\\nto 6 ft occasionally to 8 ft expected.\\n\\n* WHERE...Winthrop Harbor to Calumet Harbor IL, and Calumet\\nHarbor IL to Gary IN.\\n\\n* WHEN...For the first Small Craft Advisory, until 10 AM CST\\nthis morning. For the second Small Craft Advisory, from 9 PM\\nthis evening to 9 AM CST Thursday.\\n\\n* IMPACTS...Conditions will be hazardous to small craft.\",\n                \"instruction\": \"Inexperienced mariners, especially those operating smaller\\nvessels, should avoid navigating in hazardous conditions.\",\n                \"response\": \"Avoid\",\n                \"parameters\": {\n                    \"AWIPSidentifier\": [\n                        \"MWWLOT\"\n                    ],\n                    \"WMOidentifier\": [\n                        \"WHUS73 KLOT 030901\"\n                    ],\n                    \"NWSheadline\": [\n                        \"SMALL CRAFT ADVISORY REMAINS IN EFFECT UNTIL 10 AM CST THIS MORNING... ...SMALL CRAFT ADVISORY REMAINS IN EFFECT FROM 9 PM THIS EVENING TO 9 AM CST THURSDAY\"\n                    ],\n                    \"BLOCKCHANNEL\": [\n                        \"EAS\",\n                        \"NWEM\",\n                        \"CMAS\"\n                    ],\n                    \"VTEC\": [\n                        \"/O.CON.KLOT.SC.Y.0107.251204T0300Z-251204T1500Z/\"\n                    ],\n                    \"eventEndingTime\": [\n                        \"2025-12-04T09:00:00-06:00\"\n                    ],\n                    \"expiredReferences\": [\n                        \"w-nws.webmaster@noaa.gov,urn:oid:2.49.0.1.840.0.648f1635c62c08083c73378729536c6fc4072c7f.001.2,2025-12-02T15:03:00-06:00\"\n                    ]\n                },\n                \"scope\": \"Public\",\n                \"code\": \"IPAWSv1.0\",\n                \"language\": \"en-US\",\n                \"web\": \"http://www.weather.gov\",\n                \"eventCode\": {\n                    \"SAME\": [\n                        \"NWS\"\n                    ],\n                    \"NationalWeatherService\": [\n                        \"SCY\"\n                    ]\n                }\n            }\n        },\n        {\n            \"id\": \"https://api.weather.gov/alerts/urn:oid:2.49.0.1.840.0.dab1393c914b230290374bee41bf50b08330d8fe.002.1\",\n            \"type\": \"Feature\",\n            \"geometry\": null,\n            \"properties\": {\n                \"@id\": \"https://api.weather.gov/alerts/urn:oid:2.49.0.1.840.0.dab1393c914b230290374bee41bf50b08330d8fe.002.1\",\n                \"@type\": \"wx:Alert\",\n                \"id\": \"urn:oid:2.49.0.1.840.0.dab1393c914b230290374bee41bf50b08330d8fe.002.1\",\n                \"areaDesc\": \"Michigan Waters of Lake Erie from Detroit River to North Cape MI\",\n                \"geocode\": {\n                    \"SAME\": [\n                        \"096444\"\n                    ],\n                    \"UGC\": [\n                        \"LEZ444\"\n                    ]\n                },\n                \"affectedZones\": [\n                    \"https://api.weather.gov/zones/forecast/LEZ444\"\n                ],\n                \"references\": [\n                    {\n                        \"@id\": \"https://api.weather.gov/alerts/urn:oid:2.49.0.1.840.0.f40c017fac209f535ffd25db0b6db1cfba1965b3.001.1\",\n                        \"identifier\": \"urn:oid:2.49.0.1.840.0.f40c017fac209f535ffd25db0b6db1cfba1965b3.001.1\",\n                        \"sender\": \"w-nws.webmaster@noaa.gov\",\n                        \"sent\": \"2025-12-03T03:54:00-05:00\"\n                    },\n                    {\n                        \"@id\": \"https://api.weather.gov/alerts/urn:oid:2.49.0.1.840.0.a3167b3c58ef7b788094d623d07dc49d7b6dc5a5.001.1\",\n                        \"identifier\": \"urn:oid:2.49.0.1.840.0.a3167b3c58ef7b788094d623d07dc49d7b6dc5a5.001.1\",\n                        \"sender\": \"w-nws.webmaster@noaa.gov\",\n                        \"sent\": \"2025-12-03T03:57:00-05:00\"\n                    }\n                ],\n                \"sent\": \"2025-12-03T04:01:00-05:00\",\n                \"effective\": \"2025-12-03T04:01:00-05:00\",\n                \"onset\": \"2025-12-03T10:00:00-05:00\",\n                \"expires\": \"2025-12-03T16:15:00-05:00\",\n                \"ends\": \"2025-12-03T22:00:00-05:00\",\n                \"status\": \"Actual\",\n                \"messageType\": \"Update\",\n                \"category\": \"Met\",\n                \"severity\": \"Minor\",\n                \"certainty\": \"Likely\",\n                \"urgency\": \"Expected\",\n                \"event\": \"Low Water Advisory\",\n                \"sender\": \"w-nws.webmaster@noaa.gov\",\n                \"senderName\": \"NWS Detroit/Pontiac MI\",\n                \"headline\": \"Low Water Advisory issued December 3 at 4:01AM EST until December 3 at 10:00PM EST by NWS Detroit/Pontiac MI\",\n                \"description\": \"* WHAT...Abnormally low water levels expected.\\n\\n* WHERE...Michigan Waters of Lake Erie from Detroit River to\\nNorth Cape MI.\\n\\n* WHEN...From 10 AM this morning to 10 PM EST this evening.\\n\\n* IMPACTS...Below normal water levels will result in hazardous\\nnavigating conditions.\\n\\n* ADDITIONAL DETAILS...Elevated southwest winds through this\\nevening will result in water levels across the western basin of\\nLake Erie to fall near or slightly below the critical mark for\\nsafe navigation of 5 inches below low water datum.\",\n                \"instruction\": \"Mariners should navigate shallow waters with extreme caution due\\nto below normal water levels.\",\n                \"response\": \"Avoid\",\n                \"parameters\": {\n                    \"AWIPSidentifier\": [\n                        \"MWWDTX\"\n                    ],\n                    \"WMOidentifier\": [\n                        \"WHUS73 KDTX 030901\"\n                    ],\n                    \"NWSheadline\": [\n                        \"LOW WATER ADVISORY REMAINS IN EFFECT FROM 10 AM THIS MORNING TO 10 PM EST THIS EVENING\"\n                    ],\n                    \"BLOCKCHANNEL\": [\n                        \"EAS\",\n                        \"NWEM\",\n                        \"CMAS\"\n                    ],\n                    \"VTEC\": [\n                        \"/O.CON.KDTX.LO.Y.0011.251203T1500Z-251204T0300Z/\"\n                    ],\n                    \"eventEndingTime\": [\n                        \"2025-12-03T22:00:00-05:00\"\n                    ]\n                },\n                \"scope\": \"Public\",\n                \"code\": \"IPAWSv1.0\",\n                \"language\": \"en-US\",\n                \"web\": \"http://www.weather.gov\",\n                \"eventCode\": {\n                    \"SAME\": [\n                        \"NWS\"\n                    ],\n                    \"NationalWeatherService\": [\n                        \"LOY\"\n                    ]\n                }\n            }\n        },\n        {\n            \"id\": \"https://api.weather.gov/alerts/urn:oid:2.49.0.1.840.0.dab1393c914b230290374bee41bf50b08330d8fe.003.1\",\n            \"type\": \"Feature\",\n            \"geometry\": null,\n            \"properties\": {\n                \"@id\": \"https://api.weather.gov/alerts/urn:oid:2.49.0.1.840.0.dab1393c914b230290374bee41bf50b08330d8fe.003.1\",\n                \"@type\": \"wx:Alert\",\n                \"id\": \"urn:oid:2.49.0.1.840.0.dab1393c914b230290374bee41bf50b08330d8fe.003.1\",\n                \"areaDesc\": \"Outer Saginaw Bay SW of Alabaster to Port Austin MI to Inner Saginaw Bay; Inner Saginaw Bay SW of Point Au Gres to Bay Port MI; Port Austin to Harbor Beach MI\",\n                \"geocode\": {\n                    \"SAME\": [\n                        \"093421\",\n                        \"093422\",\n                        \"093441\"\n                    ],\n                    \"UGC\": [\n                        \"LHZ421\",\n                        \"LHZ422\",\n                        \"LHZ441\"\n                    ]\n                },\n                \"affectedZones\": [\n                    \"https://api.weather.gov/zones/forecast/LHZ421\",\n                    \"https://api.weather.gov/zones/forecast/LHZ422\",\n                    \"https://api.weather.gov/zones/forecast/LHZ441\"\n                ],\n                \"references\": [\n                    {\n                        \"@id\": \"https://api.weather.gov/alerts/urn:oid:2.49.0.1.840.0.e508fee38c3aac406abf5203bd60bd37da94117d.001.1\",\n                        \"identifier\": \"urn:oid:2.49.0.1.840.0.e508fee38c3aac406abf5203bd60bd37da94117d.001.1\",\n                        \"sender\": \"w-nws.webmaster@noaa.gov\",\n                        \"sent\": \"2025-12-02T15:41:00-05:00\"\n                    },\n                    {\n                        \"@id\": \"https://api.weather.gov/alerts/urn:oid:2.49.0.1.840.0.080b6b4f68887d4bfac38f2fc9a900ed7a28ed28.001.1\",\n                        \"identifier\": \"urn:oid:2.49.0.1.840.0.080b6b4f68887d4bfac38f2fc9a900ed7a28ed28.001.1\",\n                        \"sender\": \"w-nws.webmaster@noaa.gov\",\n                        \"sent\": \"2025-12-02T21:37:00-05:00\"\n                    },\n                    {\n                        \"@id\": \"https://api.weather.gov/alerts/urn:oid:2.49.0.1.840.0.f40c017fac209f535ffd25db0b6db1cfba1965b3.002.1\",\n                        \"identifier\": \"urn:oid:2.49.0.1.840.0.f40c017fac209f535ffd25db0b6db1cfba1965b3.002.1\",\n                        \"sender\": \"w-nws.webmaster@noaa.gov\",\n                        \"sent\": \"2025-12-03T03:54:00-05:00\"\n                    },\n                    {\n                        \"@id\": \"https://api.weather.gov/alerts/urn:oid:2.49.0.1.840.0.a3167b3c58ef7b788094d623d07dc49d7b6dc5a5.002.1\",\n                        \"identifier\": \"urn:oid:2.49.0.1.840.0.a3167b3c58ef7b788094d623d07dc49d7b6dc5a5.002.1\",\n                        \"sender\": \"w-nws.webmaster@noaa.gov\",\n                        \"sent\": \"2025-12-03T03:57:00-05:00\"\n                    }\n                ],\n                \"sent\": \"2025-12-03T04:01:00-05:00\",\n                \"effective\": \"2025-12-03T04:01:00-05:00\",\n                \"onset\": \"2025-12-03T04:01:00-05:00\",\n                \"expires\": \"2025-12-03T16:15:00-05:00\",\n                \"ends\": \"2025-12-04T16:00:00-05:00\",\n                \"status\": \"Actual\",\n                \"messageType\": \"Update\",\n                \"category\": \"Met\",\n                \"severity\": \"Minor\",\n                \"certainty\": \"Likely\",\n                \"urgency\": \"Expected\",\n                \"event\": \"Small Craft Advisory\",\n                \"sender\": \"w-nws.webmaster@noaa.gov\",\n                \"senderName\": \"NWS Detroit/Pontiac MI\",\n                \"headline\": \"Small Craft Advisory issued December 3 at 4:01AM EST until December 4 at 4:00PM EST by NWS Detroit/Pontiac MI\",\n                \"description\": \"* WHAT...Expect sustained winds up to 27 knots from the west\\nwith gusts up to 31 knots. The largest significant waves will\\nbe 6 feet with a potential maximum wave height of 8 feet.\\n\\n* WHERE...Outer Saginaw Bay SW of Alabaster to Port Austin MI to\\nInner Saginaw Bay, Inner Saginaw Bay SW of Point Au Gres to\\nBay Port 
